vi "VI Tree.vi"   [LabVIEW 2021, in "Markdown.lvlib"]
doc: "Markdown contains three sections:\n- <b>Examples</b> - Example VIs\n- <b>API</b> - Top level VIs\n- <b>SubVIs</b> - Low level VIs"
uses:
  Markdown.lvlib
  TypeDefs/Item.ctl
  SubVIs/Global.vi
types:
  T1 = typedef "Markdown.lvlib/Item.ctl" = cluster{"Name":string, "Icon":picture, "Path":path, "Title":string, "Desc":string, "ConPane":picture, "TypeString":string, "ProjectItem":string, "VI Type":enum32{"invalid VI type", "Standard VI", "Control VI", "Global VI", "Polymorphic VI", "Configuration VI", "SubSystem", "Facade VI", "Method VI", "Statechart Diagram VI"}}
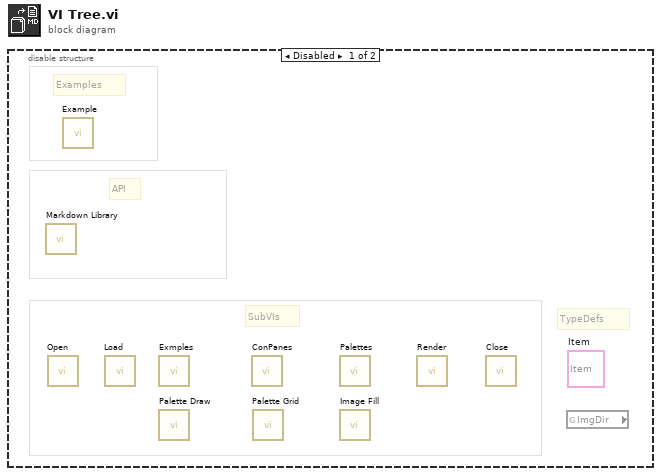
[diagram p0: block diagram]
diagram:
  n1 = disable-structure shown="Disabled" {
    frame Disabled {
      (unwired) T1 {"Name"="", "Icon"=bytes[0], "Path"=path "", "Title"="", "Desc"="", "ConPane"=bytes[0], "TypeString"="", "ProjectItem"="", "VI Type"=enum."invalid VI type"}  # Item
      # "TypeDefs"
      # "SubVIs"
      # "API"
      # "Examples"
      n2 = call "Markdown Library.vi"() -> ()  [unwired: 9 in, 3 out]
      n3 = call "Open.vi"() -> ()  [unwired: 11 in, 1 out]
      n4 = call "Example.vi"() -> ()  [unwired: 12 in]
      n5 = call "Load.vi"() -> ()  [unwired: 11 in, 1 out]
      n6 = call "Exmples.vi"() -> ()  [unwired: 11 in, 1 out]
      n7 = call "Palette Draw.vi"() -> ()  [unwired: 10 in, 2 out]
      n8 = call "ConPanes.vi"() -> ()  [unwired: 11 in, 1 out]
      n9 = call "Palette Grid.vi"() -> ()  [unwired: 10 in, 2 out]
      n10 = call "Palettes.vi"() -> ()  [unwired: 11 in, 1 out]
      n11 = call "Image Fill.vi"() -> ()  [unwired: 11 in, 1 out]
      n12 = call "Render.vi"() -> ()  [unwired: 11 in, 1 out]
      n13 = call "Close.vi"() -> ()  [unwired: 9 in, 3 out]
      n14 = global read "Global.vi" "ImgDir"() -> ()  [unwired: 1 out]
    }
    frame Enabled {
    }
  }
